vi "SetCommandValue.vi"(8 "error in (no error)":errorcluster caption="错误输入（无错误）", 10 "strValue":string, 11 "handle":u64) -> (0 "error out":errorcluster caption="错误输出", 2 "function return":i32, 3 "handle out":u64)   [LabVIEW 2011, in "MvCameraControl.lvlib"]
doc: "MV_LV_API int __stdcall SetCommandValue( void* handle, const char* strValue);"
uses:
  MvCameraControl.lvlib
  MvCameraControl.dll
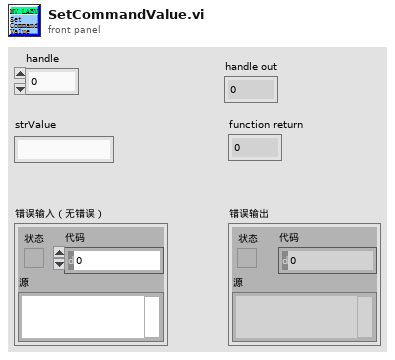
[diagram p1: front panel]
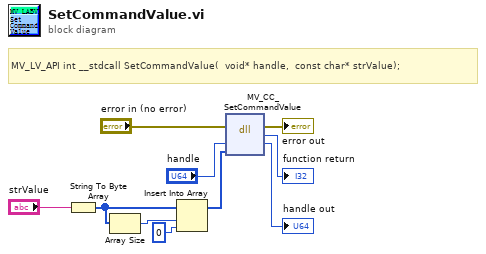
[diagram p0: block diagram]
diagram:
  # "MV_LV_API int __stdcall SetCommandValue(  void* handle,  const char* strValue);"
  n1 = String To Byte Array(string="strValue") -> (unsigned byte array=w5:u8[])
  n2 = Array Size(array=w5) -> (size(s)=w4:i32)
  n3 = Insert Into Array(array=w5, index=w4, new element=u8 0 ("新元素/子数组")) -> (w2:u8[])
  n4 = dll-call lib="MvCameraControl.dll" fn="MV_CC_SetCommandValue"(error in="error in (no error)", "handle"="handle", "strValue"=w2) -> (error out=→"error out":errorcluster, "返回类型"=→"function return":i32, "handle"=→"handle out":u64)  [unwired: 3 in, 1 out]
